vi "EventLoopInit.vi"(6 "Instance":i32) -> (0 "error out":errorcluster, 2 "Loop Name":string, 3 "Event Registration Refnum":refnum<event-registration>)   [LabVIEW 2017, in "Communication.lvlib"]
uses:
  Communication.lvlib
  MsgData.ctl
  MsgAck.ctl
  QueueRepo.Action.ctl
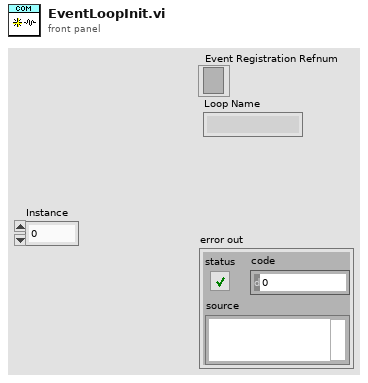
[diagram p1: front panel]
types:
  T1 = typedef "Communication.lvlib/QueueRepo.Action.ctl" = enum16{"Add", "Get", "Destroy", "Get All", "Clear"}
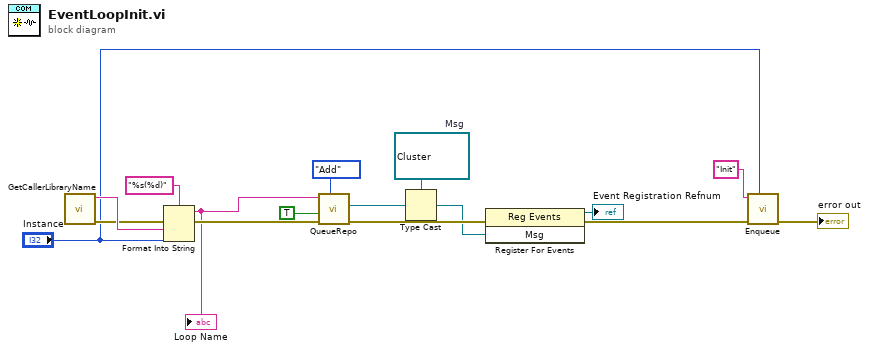
[diagram p0: block diagram]
diagram:
  w8 = refnum<user-event> refnum  # Msg
  n1 = call "GetCallerLibraryName.vi"() -> ("error out"=w14:errorcluster, "Name"=w15:string)  [unwired: 10 in]
  n2 = Format Into String(format string="%s(%d)", error in=w14, w15, "Instance") -> (resulting string=w10:string, error out=w11:errorcluster)  [unwired: 1 in]
  "Loop Name" <- w10
  n3 = call "QueueRepo.vi"("Action"=QueueRepo.Action."Add", "error in (no error)"=w11, "Event?"=TRUE, "Name"=w10) -> ("error out"=w7:errorcluster, "queue out"=w9:refnum<queue>)  [unwired: 4 in, 2 out]
  n4 = Type Cast(type=w8, x=w9) -> (*(type *) &x=w6:refnum<user-event>)
  n5 = register-events(error in=w7, w6) -> (reference out=→"Event Registration Refnum":refnum<event-registration>, error out=w4:errorcluster)  [unwired: 1 in]
  n6 = call "Enqueue.vi"("Instance"="Instance", "error in (no error)"=w4, "Msg"="Init") -> ("error out"=→"error out":errorcluster)  [unwired: 8 in]
